vi "EMV Determine Fault Code Enable.vi"(8 "error in (no error)":errorcluster, 10 "User Setpoint (0x4024) in":u16, 11 "T6 Temperature":dbl) -> (0 "error out":errorcluster, 2 "> T6+8?":bool, 3 "Disable F61?":bool)   [LabVIEW 2016]
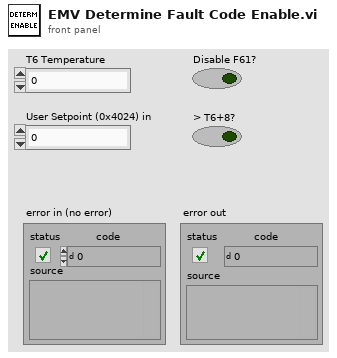
[diagram p1: front panel]
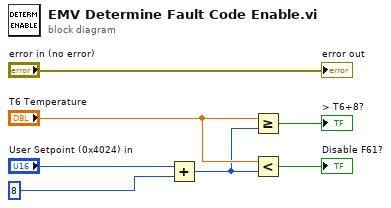
[diagram p0: block diagram]
diagram:
  n1 = Add(x="User Setpoint (0x4024) in", y=u16 8) -> (x+y=w5:u16)
  n2 = Greater Or Equal?(x="T6 Temperature", y=w5) -> (x >= y?=→"> T6+8?":bool)
  n3 = Less?(x="T6 Temperature", y=w5) -> (x < y?=→"Disable F61?":bool)
  "error out" <- "error in (no error)"
